vi "Line Configuration Dialog.vi"(8 "error in":errorcluster, 9 "engine configuration in":refnum<class "engine configuration.lvclass">, 10 "tag bus configurable plugin module configuration":refnum<class "PID Module configuration.lvclass">, 11 "Line":T2) -> (0 "error out":errorcluster, 1 "success":bool, 2 "changed":bool, 3 "Mappings out":T1)   [LabVIEW 2015, in "PID Module editor node.lvclass"]
doc: "A dialog for allowing a user to specify the values of a new line."
uses:
  PID Module editor node.lvclass
  module/configuration/Line.ctl
  <vilib>/NI/Tag Bus Module Framework/channel/TBM channel.lvclass
  Mappings.ctl
  Map.ctl
  <vilib>/NI/Module Execution Interface/Engine Configuration/engine configuration.lvclass
  module/configuration/PID Module configuration.lvclass
  <vilib>/NI/Tag Bus/tag/tag descriptor.lvclass/tag descriptor.ctl
  <vilib>/NI/Tag Bus Module Framework/channel/TBM channel.lvclass/TBM channel.ctl
  <vilib>/NI/Configuration Framework/serializable configuration/NISE_CEF_serializable configuration.lvclass/NISE_CEF_serializable configuration.ctl
  <vilib>/NI/Tag Bus/tag/write tag name.vi
  <vilib>/NI/Configuration Framework/serializable configuration/Read UID.vi
  <vilib>/NI/Tag Bus Module Framework/channel/Read channel classification.vi
  <vilib>/Utility/LVClass/Get LV Class Name.vi
  <vilib>/NI/Configuration Framework/error generator/NISE_error generator.vi
  <vilib>/NI/Tag Bus/tag/tag descriptor.lvclass
  <vilib>/NI/DCAF UI Toolkit/Controls/DCAF UI Elements.lvlib
panel:
  out "errors":string
  in  "Tag":i32(listbox)
  in  "PID Id":string
  in  "cancel":bool
  in  "ok":bool
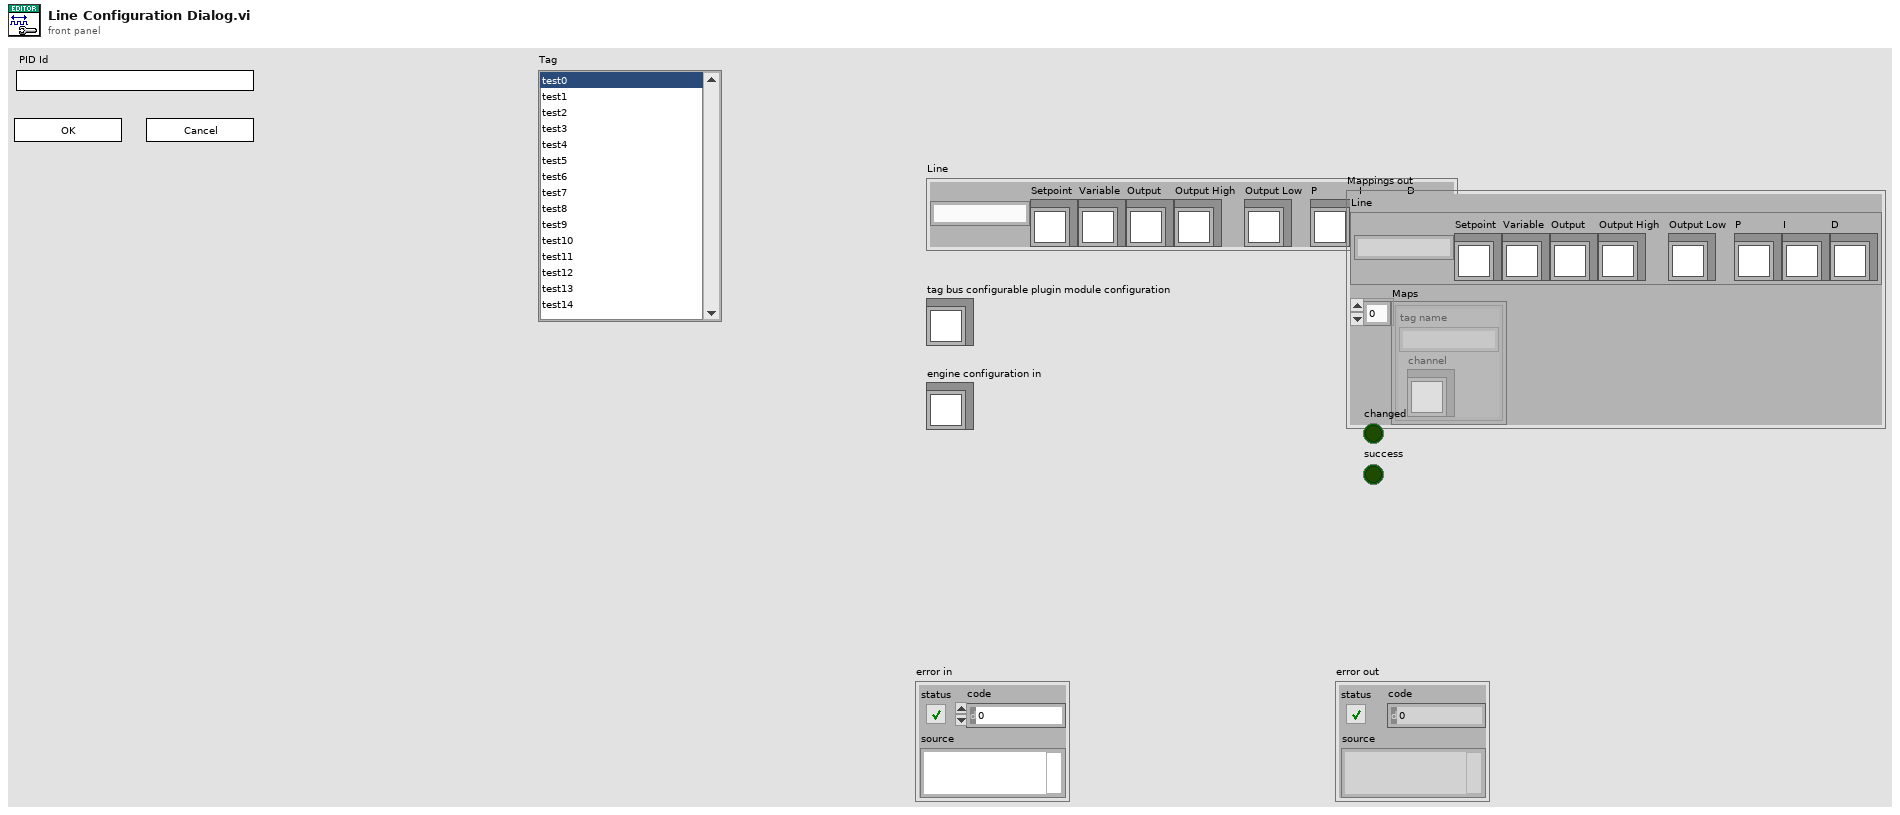
[diagram p1: front panel]
types:
  T1 = typedef "PID Module editor node.lvclass/Mappings.ctl" = cluster{"Line":T2, "Maps":T3[]}
  T2 = typedef "PID Module configuration.lvclass/Line.ctl" = cluster{"PID ID":string, "Setpoint":refnum<class "TBM channel.lvclass">, "Variable":refnum<class "TBM channel.lvclass">, "Output":refnum<class "TBM channel.lvclass">, "Output High":refnum<class "TBM channel.lvclass">, "Output Low":refnum<class "TBM channel.lvclass">, "P":refnum<class "TBM channel.lvclass">, "I":refnum<class "TBM channel.lvclass">, "D":refnum<class "TBM channel.lvclass">}
  T3 = typedef "PID Module editor node.lvclass/Map.ctl" = cluster{"channel":refnum<class "TBM channel.lvclass">, "tag name":string}
  T4 = typedef "TBM channel.lvclass/channel classification.ctl" = enum16{"input data", "output data", "processing parameter", "processing result"}
  T5 = enum8{"Enabled", "Disabled", "Disabled and Grayed Out"}
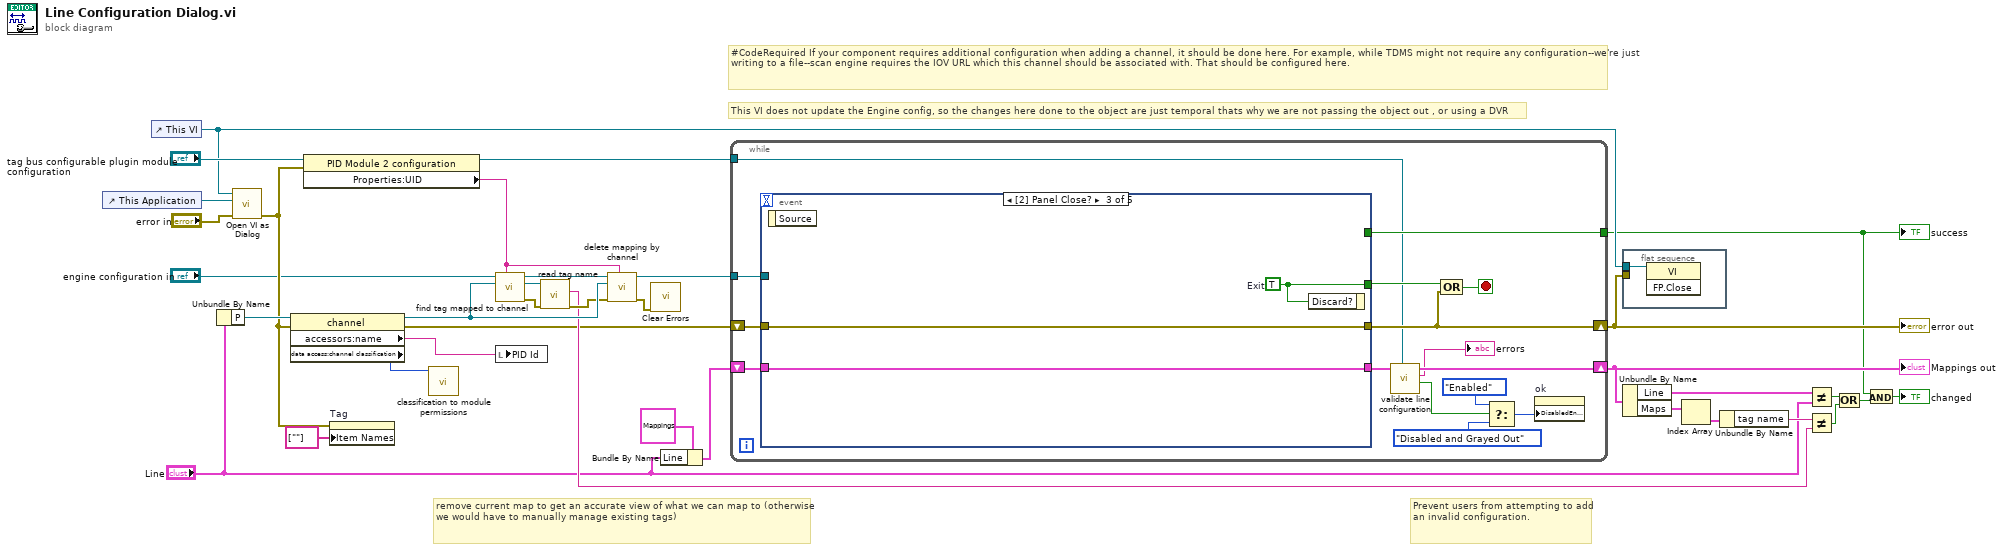
[diagram p0: block diagram]
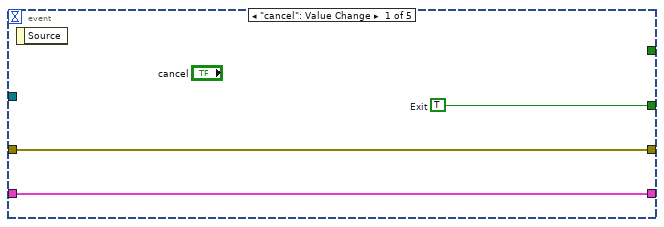
[diagram p2: hidden frame]
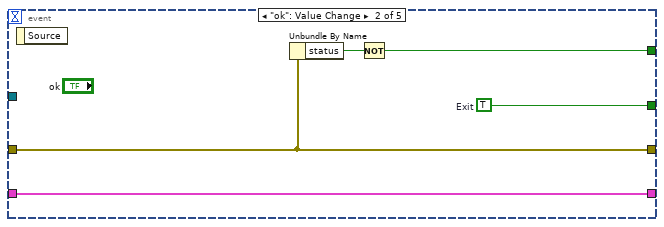
[diagram p3: hidden frame]
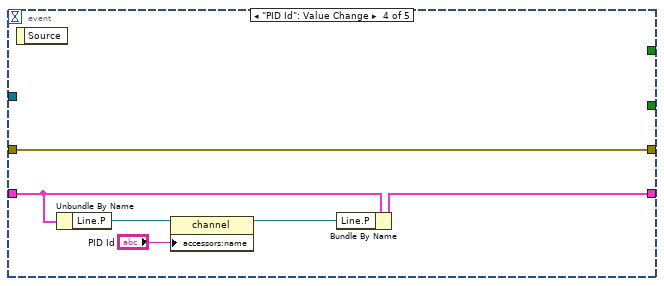
[diagram p4: hidden frame]
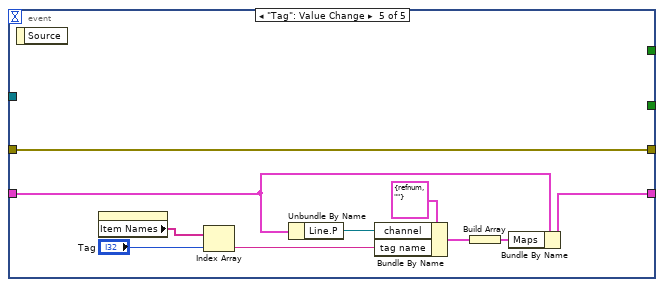
[diagram p5: hidden frame]
diagram:
  # "Prevent users from attempting to add an invalid configuration."
  # "This VI does not update the Engine config, so the changes here done to the object are just temporal thats why we are not passing the object out , or using a DVR"
  # "remove current map to get an accurate view of what we can map to (otherwise we would have to manually manage existing tags)"
  # "#CodeRequired If your component requires additional configuration when adding a channel, it should be done here. For example, while TDMS might not require any configuration--we're just writing to a file--scan engine requires the IOV URL which this channel should be associated with. That should be configured here."
  n1 = control-ref of="This Application"() -> (w26:refnum<vi>)
  n2 = control-ref of="This VI"() -> (w11:refnum<vi>)
  n3 = Unbundle By Name("Line") -> ("P"=w34:refnum<class "TBM channel.lvclass">)
  n4 = call <vilib>:"Open VI as Dialog.vi"("error in (no error)"="error in", "This Application"=w26, "VI in"=w11) -> ("error out"=w24:errorcluster)  [unwired: 8 in]
  n5 = property class="channel"(reference=w34, error in=w24) -> (reference out=w20:refnum<class "TBM channel.lvclass">, error out=w6:errorcluster, "accessors:name"=w5:string, "data access:channel classification"=w7:T4)
  n6 = property class="PID Module 2 configuration"(reference="tag bus configurable plugin module configuration", error in=w24) -> (reference out=w21:refnum<class "PID Module configuration.lvclass">, "Properties:UID"=w8:string)  [unwired: 1 out]
  n7 = property on="Tag" class="LstBox (strict)"(error in=w24, "Item Names"=string[] [""]) -> ()  [unwired: 1 in, 2 out]
  n8 = call "classification to module permissions.vi"("channel classification"=w7) -> ()  [unwired: 10 in, 1 out]
  n9 = call <vilib>:"find tag mapped to channel.vi"("owner"=w8, "channel"=w20, "engine configuration in"="engine configuration in") -> ("error out"=w18:errorcluster, "tag"=w19:refnum<class "tag descriptor.lvclass">, "engine configuration out"=w22:refnum<class "engine configuration.lvclass">)  [unwired: 6 in]
  n10 = local write "PID Id"(w5) -> ()
  n11 = call <vilib>:"read tag name.vi"("error in"=w18, "system tag in"=w19) -> ("error out"=w17:errorcluster, "name"=w10:string)  [unwired: 7 in, 1 out]
  n12 = call <vilib>:"delete mapping by channel.vi"("owner ID"=w8, "error in"=w17, "channel"=w20, "engine configuration in"=w22) -> ("error out"=w32:errorcluster, "engine configuration out"=w35:refnum<class "engine configuration.lvclass">)  [unwired: 6 in]
  n13 = call <vilib>:"Clear Errors.vi"("error in (no error)"=w32) -> ()  [unwired: 5 in, 2 out]
  n14 = Bundle By Name(cluster=T1 {"Line"={"PID ID"="", "Setpoint"=refnum, "Variable"=refnum, "Output"=refnum, "Output High"=refnum, "Output Low"=refnum, "P"=refnum, "I"=refnum, "D"=refnum}, "Maps"=[]} ("Mappings out"), "Line"="Line") -> (w29:T1)
  n15 = while {
    shift-right: [w42] -> w4
    shift-left: w6 -> [w49]
    tunnel: [w48] -> w3
    shift-right: [w43] -> w27
    shift-left: w29 -> [w45]
    tunnel: w35 -> [w50]
    tunnel: w21 -> [w37]
    stop <- w46 stop-if-true
    n16 = event shown="[2] Panel Close?" {
      selector: _ -> [_ _ _ _ _]
      dyn-events: _ -> [_ _ _ _ _]
      timeout: _ -> [_ _ _ _ _]
      tunnel: w50 -> [_ _ _ _ _]
      tunnel: w49 -> [w53 w56 w61 w67 w77]
      tunnel: [w53 w56 w61 w67 w77] -> w42
      tunnel: [_ w54 _ _ _] -> w48
      tunnel: [w51 w57 w59 _ _] -> w47
      tunnel: w45 -> [w52 w58 w60 w65 w68]
      tunnel: [w52 w58 w60 w66 w70] -> w44
      event "cancel": Value Change {
        w51 = TRUE  # Exit
        n17 = event-data() -> ()  [unwired: 1 in, 1 out]
      }
      event "ok": Value Change {
        w57 = TRUE  # Exit
        n18 = event-data() -> ()  [unwired: 1 in, 1 out]
        n19 = Unbundle By Name(w56) -> ("status"=w55:bool)
        n20 = Not(x=w55) -> (.not. x?=w54:bool)
      }
      event Panel Close? {
        w59 = TRUE  # Exit
        n21 = event-data() -> ()  [unwired: 1 in, 1 out]
        n22 = event-data("Discard?"=w59) -> ()  [unwired: 1 in, 1 out]
      }
      event "PID Id": Value Change {
        n23 = event-data() -> ()  [unwired: 1 in, 1 out]
        n24 = Unbundle By Name(w65) -> ("Line.P"=w64:refnum<class "TBM channel.lvclass">)
        n25 = property class="channel"(reference=w64, "accessors:name"="PID Id") -> (reference out=w63:refnum<class "TBM channel.lvclass">)  [unwired: 1 in, 1 out]
        n26 = Bundle By Name(cluster=w65, "Line.P"=w63) -> (w66:T1)
      }
      event "Tag": Value Change {
        n27 = event-data() -> ()  [unwired: 1 in, 1 out]
        n28 = property on="Tag" class="LstBox (strict)"() -> ("Item Names"=w75:string[])  [unwired: 2 in, 2 out]
        n29 = Index Array(array=w75, index="Tag") -> (element=w69:string)
        n30 = Unbundle By Name(w68) -> ("Line.P"=w73:refnum<class "TBM channel.lvclass">)
        n31 = Bundle By Name(cluster=T3 {"channel"=refnum, "tag name"=""} ("Map"), "channel"=w73, "tag name"=w69) -> (w72:T3)
        n32 = Build Array(w72) -> (w71:T3[])
        n33 = Bundle By Name(cluster=w68, "Maps"=w71) -> (w70:T1)
      }
    }
    n34 = call "validate line configuration.vi"("Module Config"=w37, "Mappings in"=w44) -> ("valid?"=w41:bool, "errors"=→"errors":string, "Mappings out"=w43:T1)  [unwired: 7 in]
    n35 = Compound Arithmetic op=OR(w47, w42) -> (w46:bool)
    n36 = Select(t=T5."Enabled" ("Disabled"), s=w41, f=T5."Disabled and Grayed Out") -> (s? t:f=w38:T5)
    n37 = property on="ok" class="Bool"("DisabledEnum"=w38) -> ()  [unwired: 2 in, 2 out]
  }
  "error out" <- w4
  "success" <- w3
  "Mappings out" <- w27
  n38 = flat-sequence {
    tunnel: w4 -> [_]
    tunnel: w11 -> [w78]
    frame #0 {
      n39 = invoke class="VI" method="FP.Close"(reference=w78) -> ()  [unwired: 2 in, 3 out]
    }
  }
  n40 = Unbundle By Name(w27) -> ("Line"=w28:T2, "Maps"=w16:T3[])
  n41 = Index Array(array=w16) -> (element=w15:T3)  [unwired: 1 in]
  n42 = Unbundle By Name(w15) -> ("tag name"=w14:string)
  n43 = Not Equal?(x=w28, y="Line") -> (x != y?=w12:bool)
  n44 = Not Equal?(x=w14, y=w10) -> (x != y?=w13:bool)
  n45 = Or(x=w12, y=w13) -> (x .or. y?=w2:bool)
  n46 = And(x=w3, y=w2) -> (x .and. y?=→"changed":bool)
